vi "Set APSVG parameters.vi"(0 "Signal generator configuration":T2={"Lower limit [GHz]"=0.0, "Upper limit [GHz]"=20.0, "Device name"="VDIYT7", "Connection"="", "Description"="VDI Tracking", "Connected"=FALSE, "Last settings"="", "Operation mode"=enum."Disabled", "Enable ch 1"=FALSE, "Enable ch 2"=FALSE}, 9 "Sweep parameters":T1 {"Sweep down\ntime [ms]" min=0.0 max=250.0; "End [GHz]" min=0.0 max=20.0; "Intermidiate [MHz]" min=0.0 max=2500.0; "Start [GHz]" min=0.0 max=20.0}) -> (4 "Signal generator configuration out":T2={"Lower limit [GHz]"=8.0, "Upper limit [GHz]"=20.0, "Device name"="VDIYT7", "Connection"="", "Description"="VDI Tracking", "Connected"=FALSE, "Last settings"="", "Operation mode"=enum."Disabled", "Enable ch 1"=FALSE, "Enable ch 2"=FALSE}, 10 "Sweep parameters out":T1={"Start [GHz]"=8.0, "End [GHz] "=8.0, "Sweep up\ntime [ms]"=0.0, "Sweep down\ntime [ms]"=0.0, "Intermidiate [MHz]"=0.0, "Reset trigger"=FALSE} {"Sweep down\ntime [ms]" min=0.0 max=250.0; "End [GHz]" min=8.0 max=20.0; "Intermidiate [MHz]" min=0.0 max=2500.0; "Start [GHz]" min=8.0 max=20.0}, 15 "error out":errorcluster)   [LabVIEW 2024, in "THz source modeule.lvlib"]
uses:
  THz source modeule.lvlib
  ctl/THz sweep parameters.ctl
  ctl/THz MW generator constants.ctl
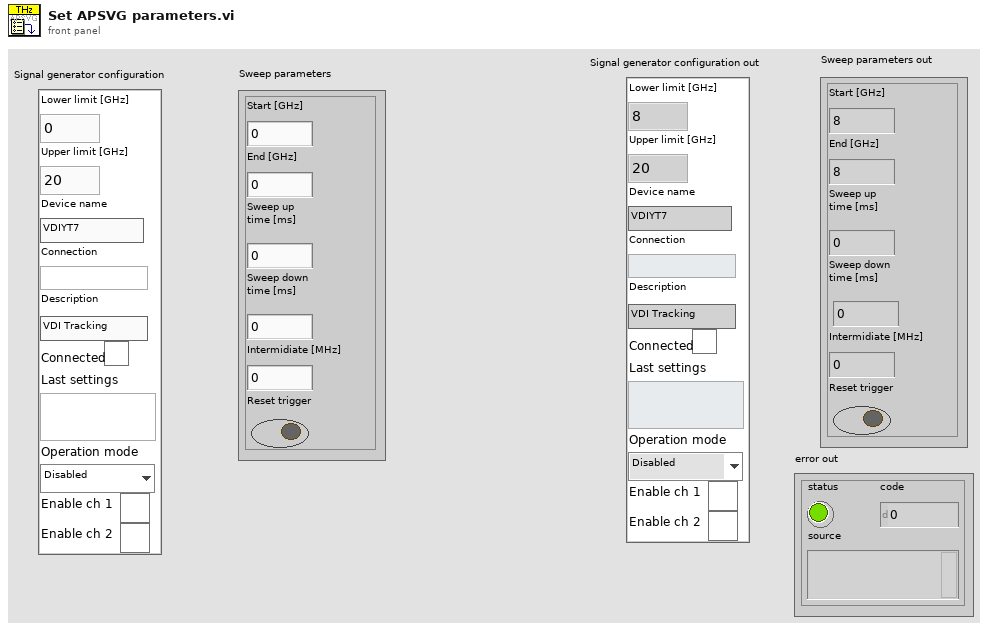
[diagram p1: front panel]
types:
  T1 = typedef "THz source modeule.lvlib/THz sweep parameters.ctl" = cluster{"Start [GHz]":dbl, "End [GHz] ":dbl, "Sweep up\ntime [ms]":dbl, "Sweep down\ntime [ms]":dbl, "Intermidiate [MHz]":dbl, "Reset trigger":bool}
  T2 = typedef "THz source modeule.lvlib/THz MW generator constants.ctl" = cluster{"Lower limit [GHz]":dbl, "Upper limit [GHz]":dbl, "Device name":string, "Connection":string, "Description":string, "Connected":bool, "Last settings":string, "Operation mode":enum16{"Disabled", "CW", "Arbitrary", "Sweep"}, "Enable ch 1":bool, "Enable ch 2":bool}
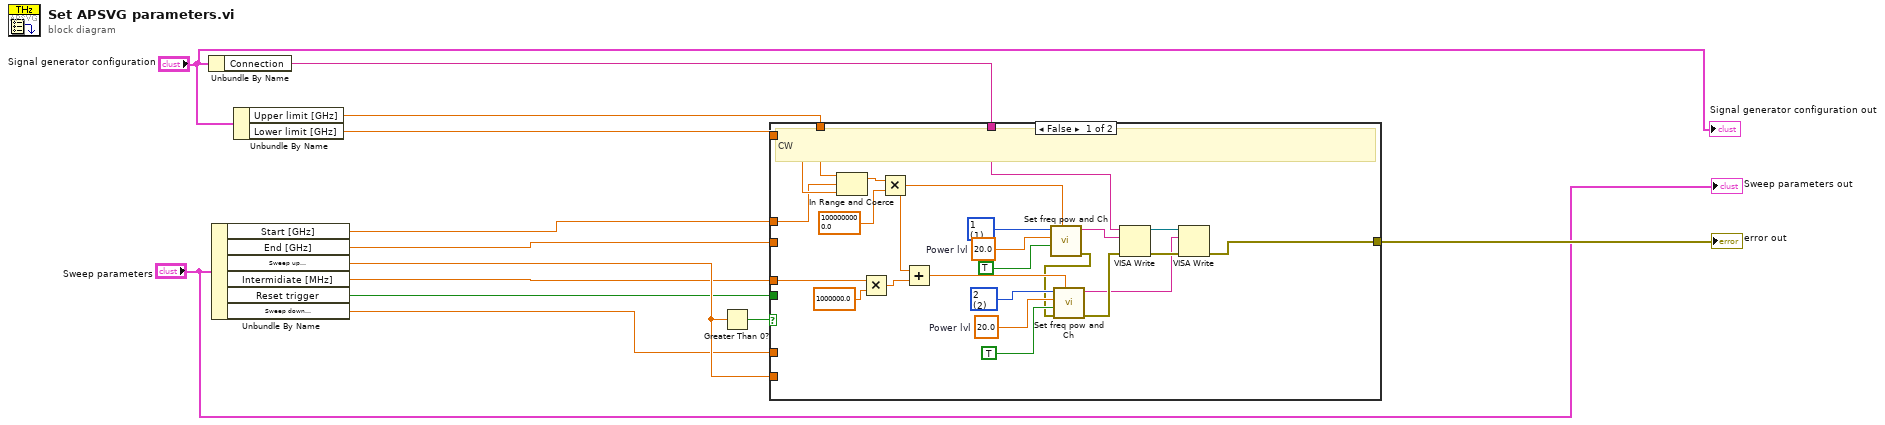
[diagram p0: block diagram]
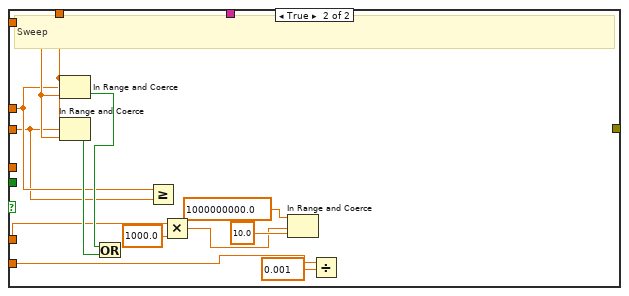
[diagram p2: hidden frame]
diagram:
  n1 = Unbundle By Name("Signal generator configuration") -> ("Connection"=w5:string)
  n2 = Unbundle By Name("Sweep parameters") -> ("Start [GHz]"=w7:dbl, "End [GHz]"=w12:dbl, "Sweep up\ntime [ms]"=w9:dbl, "Intermidiate [MHz]"=w6:dbl, "Reset trigger"=w1:bool, "Sweep down\ntime [ms]"=w8:dbl)
  n3 = Unbundle By Name("Signal generator configuration") -> ("Upper limit [GHz]"=w13:dbl, "Lower limit [GHz]"=w11:dbl)
  n4 = Greater Than 0?(x=w9) -> (x > 0?=w10:bool)
  n5 = case shown="False" w10 {
    tunnel: w7 -> [w35 w45]
    tunnel: w11 -> [w36 w50]
    tunnel: w12 -> [_ w44]
    tunnel: w13 -> [w37 w49]
    tunnel: w9 -> [_ w43]
    tunnel: w8 -> [_ w42]
    tunnel: w6 -> [w33 _]
    tunnel: w5 -> [w17 _]
    tunnel: [w16 _] -> w3
    tunnel: w1 -> [_ _]
    frame False {
      w26 = 20.0  # Power lvl
      w25 = 2 items=["1"=1, "2"=2] ("Channel")
      w30 = 20.0  # Power lvl
      w31 = 1 items=["1"=1, "2"=2] ("Channel")
      # "CW"
      n6 = In Range and Coerce(upper limit=w37, x=w35, lower limit=w36) -> (coerced(x)=w28:dbl)  [unwired: 1 out]
      n7 = Multiply(x=w33, y=1000000.0) -> (x*y=w34:dbl)
      n8 = Multiply(x=w28, y=1000000000.0) -> (x*y=w15:dbl)
      n9 = Add(x=w15, y=w34) -> (x+y=w24:dbl)
      n10 = call "Set freq pow and Ch.vi"("Frequency Hz"=w15, "On/Off"=TRUE, "Power lvl"=w30, "Channel"=w31) -> ("error out"=w23:errorcluster, "resulting string"=w21:string)  [unwired: 6 in]
      n11 = call "Set freq pow and Ch.vi"("Frequency Hz"=w24, "error in (no error)"=w23, "On/Off"=TRUE, "Power lvl"=w26, "Channel"=w25) -> ("error out"=w22:errorcluster, "resulting string"=w18:string)  [unwired: 5 in]
      n12 = VISA Write(VISA resource name=w17, write buffer=w21, error in (no error)=w22) -> (VISA resource name out=w19:refnum<visa-resource-name>, error out=w20:errorcluster)  [unwired: 1 out]
      n13 = VISA Write(VISA resource name=w19, write buffer=w18, error in (no error)=w20) -> (error out=w16:errorcluster)  [unwired: 2 out]
    }
    frame True {
      # "Sweep"
      n14 = In Range and Coerce(upper limit=w49, x=w45, lower limit=w50) -> (In Range?=w48:bool)  [unwired: 1 out]
      n15 = In Range and Coerce(upper limit=w49, x=w44, lower limit=w50) -> (In Range?=w47:bool)  [unwired: 1 out]
      n16 = Or(x=w48, y=w47) -> ()  [unwired: 1 out]
      n17 = Greater Or Equal?(x=w45, y=w44) -> ()  [unwired: 1 out]
      n18 = Multiply(x=w42, y=1000.0 ("Sweep down\ntime [ms]")) -> (x*y=w39:dbl)
      n19 = In Range and Coerce(upper limit=1000000000.0, x=w39, lower limit=10.0) -> ()  [unwired: 2 out]
      n20 = Divide(x=w43, y=0.001) -> ()  [unwired: 1 out]
    }
  }
  "error out" <- w3
  "Signal generator configuration out" <- "Signal generator configuration"
  "Sweep parameters out" <- "Sweep parameters"
